vi "test_Remove Speciality Input Channel.vi"(8 "error in (no error)":errorcluster, 11 "TestCase in":refnum<class "FPGA Addon Adding a Channel Item.lvclass">) -> (0 "error out":errorcluster, 3 "TestCase out":refnum<class "FPGA Addon Adding a Channel Item.lvclass">)   [LabVIEW 2019, in "FPGA Addon Adding a Channel Item.lvclass"]
uses:
  FPGA Addon Adding a Channel Item.lvclass
  Addon/Addon Shared/Types/FG Action.ctl
  FPGA Addon Adding a Channel Item.lvclass/FPGA Addon Adding a Channel Item.ctl
  Addon/Addon Shared/SubVIs/Constants.vi
  <vilib>/NI VeriStand/Custom Device Tools/Custom Device Utility Library/NI VeriStand - Search for Item by GUID.vi
  <vilib>/NI/NI VeriStand Advanced SysDef API/SysDef API/SysDef.Property.Get.vi
  <vilib>/NI/NI VeriStand Advanced SysDef API/_SubVIs/SysDef.Property.Get.Variant.vi
  <vilib>/NI/NI VeriStand Advanced SysDef API/SysDef API/SysDef.Property.Set.vi
  <vilib>/NI/NI VeriStand Advanced SysDef API/_SubVIs/SysDef.Property.Set.Variant.vi
  <vilib>/NI/NI VeriStand Advanced SysDef API/_SubVIs/SysDef.Search.GUIDs.vi
  <vilib>/addons/_JKI Toolkits/VI Tester/TestCase.llb/TestCase.lvclass
  Addon/Addon System Explorer/FPGA Addon System Explorer.lvlib
  Addon/Addon Shared/FPGA Addon Shared.lvlib
  <vilib>/NI VeriStand/Custom Device Tools/Custom Device Utility Library/Custom Device Utility Library.lvlib
  <vilib>/NI/NI VeriStand Advanced SysDef API/SysDef API/Advanced System Definition.lvlib
  C:/Program Files (x86)/National Instruments/LabVIEW 2019/vi.lib/addons/_JKI Toolkits/VI Tester/TestCase.llb/TestCase.lvclass
panel:
  out "GUIDs":string[](array[string])
  in  "remove":bool
  in  "add":bool
  out "Names":string[](array[string])
  in  "Available Registers":i32[](listbox)
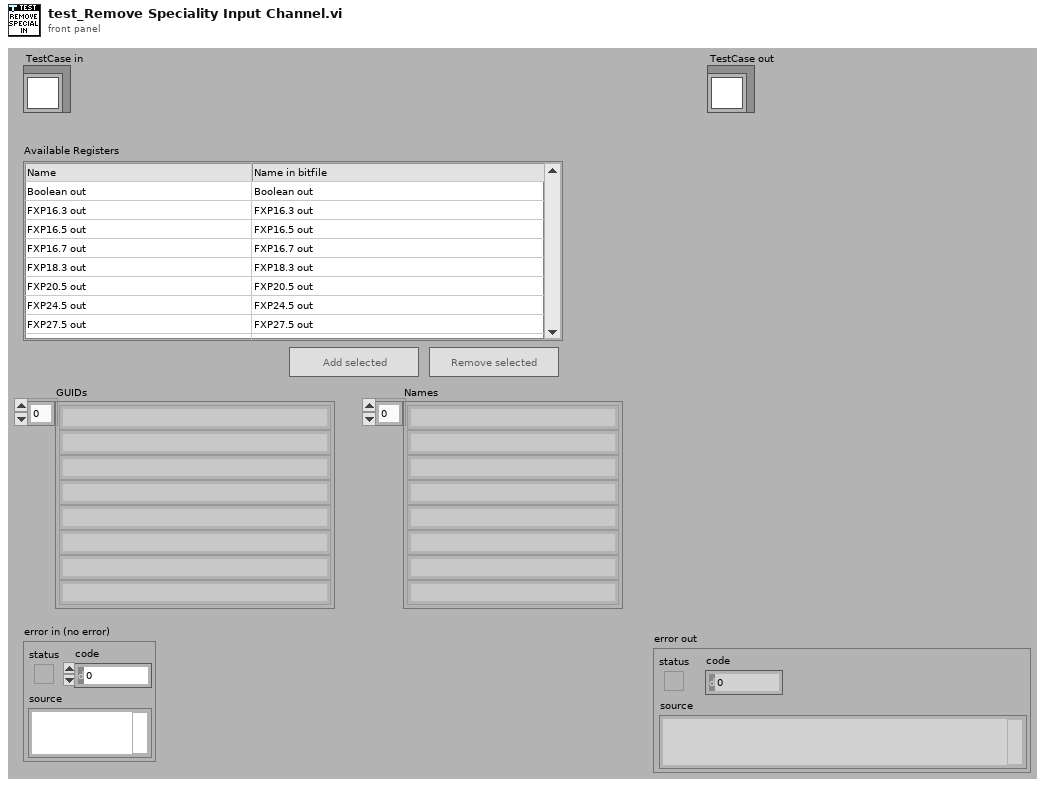
[diagram p1: front panel]
types:
  T1 = typedef "FPGA Addon Shared.lvlib/FG Action.ctl" = enum8{"GET", "SET"}
  T2 = typedef "Custom Device API.lvlib/Custom Device Item Ref.ctl" = u64
  T3 = typedef "FPGA Addon Shared.lvlib/Register Information.ctl" = cluster{"Name":string, "Data Type":T4, "Default Value":variant}
  T4 = typedef "FPGA Addon Shared.lvlib/Data Type.ctl" = enum8{"<Null>", "I8", "I16", "I32", "I64", "U8", "U16", "U32", "U64", "SGL", "Boolean", "Analog PWM In Settings", "Analog PWM In", "Digital PWM In Settings", "Digital PWM In", "Digital PWM Out", "Sine Out", "FXP+/-24.5", "FXP+/-16.5", "FXP+/-32.8", "FXP+/-64.32", "FXP+/-16.7", "FXP+/-20.5", "FXP+/-27.5", "FXP+/-32.16", "FXP+16.3", "FXP+18.3", "Digital Static In", "Digital Static Out", "Digital Static In Settings", "Digital WSS Out", "Quad Encoder Settings", "Quad Encoder In", "Group"}
  T5 = typedef "FPGA Addon System Explorer.lvlib/Listbox Cluster.ctl" = cluster{"add":refnum<vi>, "remove":refnum<vi>, "Listbox":refnum<vi>, "selected":i32[], "not present":i32[], "listbox text":string[][], "Section Ref":T2}
  T6 = typedef "Advanced System Definition.lvlib/TreeItem.Info.ctl" = cluster{"Name":string, "Description":string, "GUID":string, "Is Channel":bool, "Channel":T7, "Is Waveform":bool, "Waveform":T9}
  T7 = typedef "Custom Device API.lvlib/Custom Device Channel.ctl" = cluster{"Type":T8, "Units":string, "Default Value":dbl, "Faultable":bool, "Scalable":bool}
  T8 = typedef "Custom Device API.lvlib/Custom Device Channel Type.ctl" = enum16{"Input", "Output"}
  T9 = typedef "Custom Device API.lvlib/Custom Device Waveform.ctl" = cluster{"Data Type":T10, "Units":string}
  T10 = typedef "Custom Device API.lvlib/Custom Device Waveform DataType.ctl" = enum16{"Double", "Complex Double"}
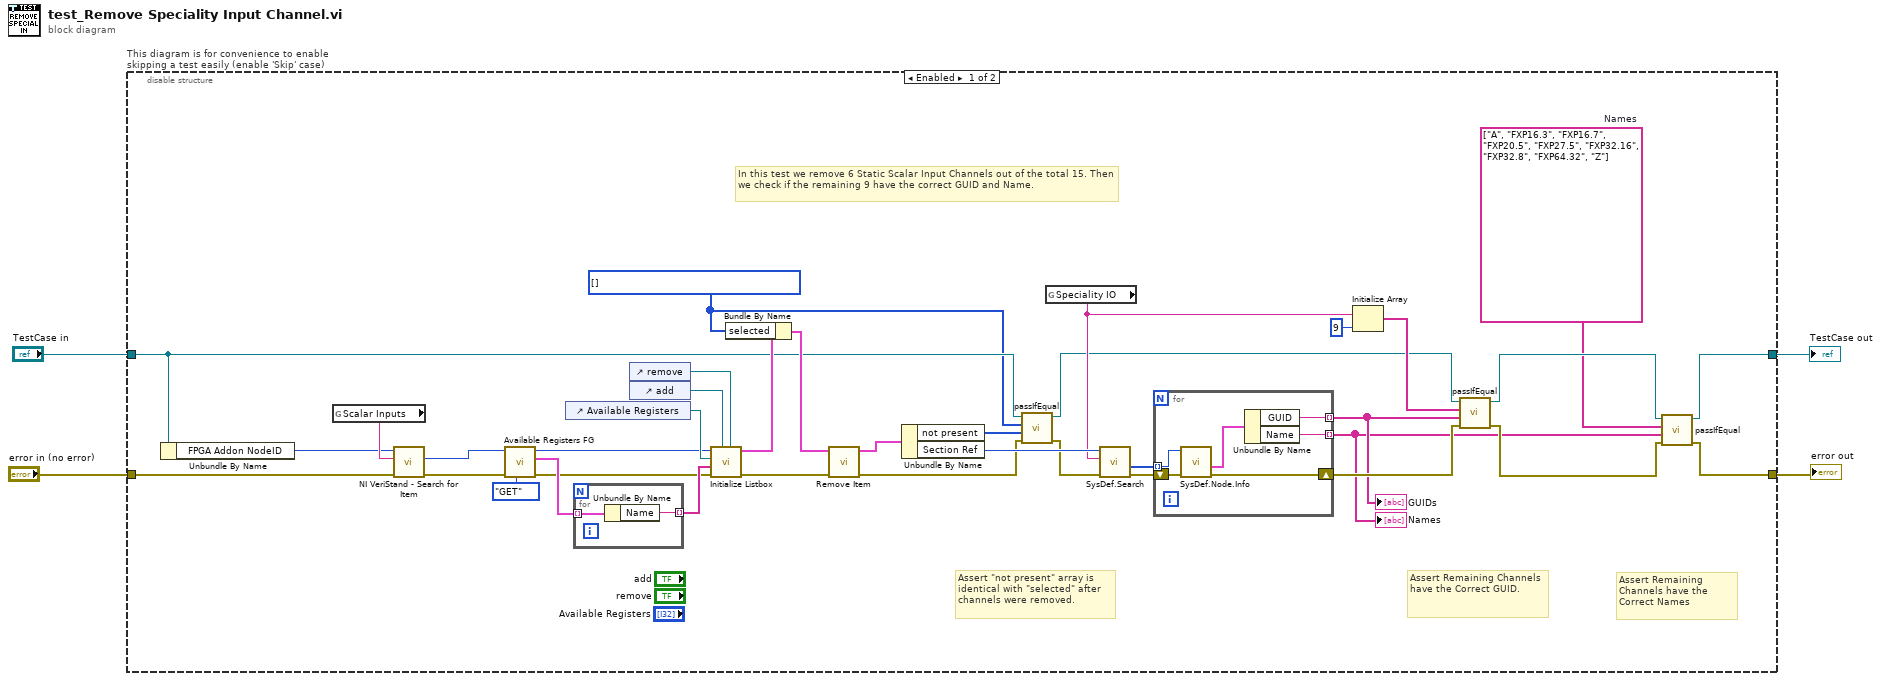
[diagram p0: block diagram]
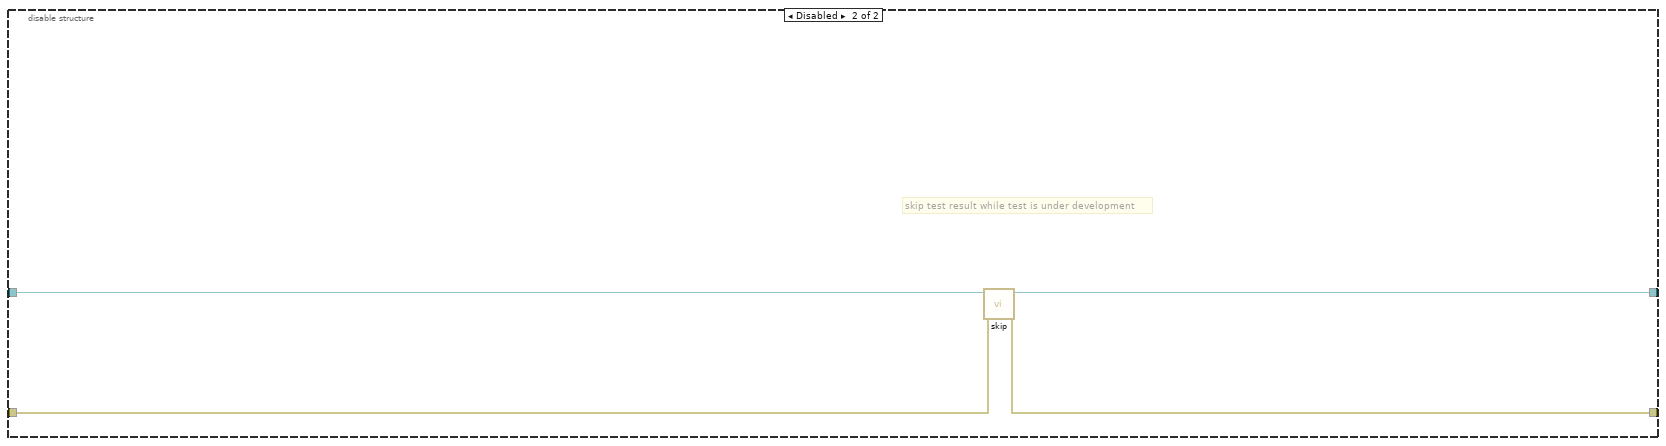
[diagram p2: hidden frame]
diagram:
  n1 = disable-structure "This diagram is for convenience to enable skipping a test easily (enable 'Skip' case)" shown="Enabled" {
    disable-tunnel: "TestCase in" -> [w7 w53]
    disable-tunnel: [w20 w51] -> w1
    disable-tunnel: [w19 w52] -> w3
    disable-tunnel: "error in (no error)" -> [w18 w50]
    frame Enabled {
      w21 = string[] ["A", "FXP16.3", "FXP16.7", "FXP20.5", "FXP27.5", "FXP32.16", "FXP32.8", "FXP64.32", "Z"]  # Names
      w5 = i32[] [] ("selected")
      # "Assert \"not present\" array is identical with \"selected\" after channels were removed."
      # "In this test we remove 6 Static Scalar Input Channels out of the total 15. Then we check if the remaining 9 have the correct GUID and Name."
      # "Assert Remaining Channels have the Correct Names"
      # "Assert Remaining Channels have the Correct GUID."
      n2 = Unbundle By Name(w7) -> ("FPGA Addon NodeID"=w17:u64)
      n3 = global read "Constants.vi" "Scalar Inputs"() -> (w36:string)
      n4 = call-poly <vilib>:"NI VeriStand - Search for Item.vi"("error in"=w18, "Item GUID"=w36, "Section Ref in"=w17) -> ("error out"=w35:errorcluster, "Item Ref"=w31:T2)  [unwired: 5 in, 2 out]
      n5 = call "Available Registers FG.vi"("Action"=FG_Action."GET", "error in (no error)"=w35, "Item Ref"=w31) -> ("error out"=w34:errorcluster, "Available Registers"=w39:T3[], "Item Ref out"=w33:T2)  [unwired: 6 in]
      n6 = control-ref of="Available Registers"() -> (w41:refnum<vi>)
      n7 = for {
        tunnel: w39 -> [w43] mode=indexing
        tunnel: [w42] -> w38 mode=indexing
        n8 = Unbundle By Name(w43) -> ("Name"=w42:string)
      }
      n9 = control-ref of="remove"() -> (w28:refnum<vi>)
      n10 = control-ref of="add"() -> (w29:refnum<vi>)
      n11 = call "Initialize Listbox.vi"("remove"=w28, "add"=w29, "error in (no error)"=w34, "Names"=w38, "Listbox"=w41, "Item Ref"=w33) -> ("error out"=w13:errorcluster, "Listbox Refs"=w37:T5)  [unwired: 4 in]
      n12 = Bundle By Name(cluster=w37, "selected"=w5) -> (w14:T5)
      n13 = call "Remove Item.vi"("error in (no error)"=w13, "Listbox Refs in"=w14) -> ("error out"=w10:errorcluster, "Listbox Refs out"=w12:T5)  [unwired: 8 in]
      n14 = Unbundle By Name(w12) -> ("not present"=w8:i32[], "Section Ref"=w30:T2)
      n15 = call-dynamic "passIfEqual.vi"("error in (no error)"=w10, "y"=w8, "x"=w5, "TestCase in"=w7) -> ("error out"=w9:errorcluster, "TestCase out"=w6:refnum<class "FPGA Addon Adding a Channel Item.lvclass">)  [unwired: 6 in]
      n16 = global read "Constants.vi" "Speciality IO"() -> (w15:string)
      n17 = call-poly <vilib>:"SysDef.Search.vi"("error in (no error)"=w9, "GUID"=w15, "nodeID"=w30) -> ("error out"=w32:errorcluster, "Values Out"=w27:u64[])  [unwired: 5 in, 2 out]
      n18 = for {
        tunnel: w27 -> [w46] mode=indexing
        tunnel: [w44] -> w22 mode=indexing
        tunnel: [w45] -> w24 mode=indexing
        shift-right: [w48] -> w25
        shift-left: w32 -> [w49]
        n19 = call <vilib>:"SysDef.Node.Info.vi"("error in (no error)"=w49, "nodeID"=w46) -> ("error out"=w48:errorcluster, "Item Info"=w47:T6)  [unwired: 6 in, 2 out]
        n20 = Unbundle By Name(w47) -> ("GUID"=w45:string, "Name"=w44:string)
      }
      "Names" <- w22
      "GUIDs" <- w24
      n21 = Initialize Array(w15, 9 ("dimension size")) -> (w16:string[])
      n22 = call-dynamic "passIfEqual.vi"("error in (no error)"=w25, "y"=w24, "x"=w16, "TestCase in"=w6) -> ("error out"=w26:errorcluster, "TestCase out"=w23:refnum<class "FPGA Addon Adding a Channel Item.lvclass">)  [unwired: 6 in]
      n23 = call-dynamic "passIfEqual.vi"("error in (no error)"=w26, "y"=w22, "x"=w21, "TestCase in"=w23) -> ("error out"=w19:errorcluster, "TestCase out"=w20:refnum<class "FPGA Addon Adding a Channel Item.lvclass">)  [unwired: 6 in]
    }
    frame Disabled {
      # "skip test result while test is under development"
      n24 = call <vilib>:"skip.vi"("error in (no error)"=w50, "TestCase in"=w53) -> ("error out"=w52:errorcluster, "TestCase out"=w51:refnum<class "FPGA Addon Adding a Channel Item.lvclass">)  [unwired: 8 in]
    }
  }
  "error out" <- w3
  "TestCase out" <- w1
